vi "Accel Distance Calculator.vi"(11 "G-Input":dbl) -> (3 "Distance gone":dbl)   [LabVIEW 2014]
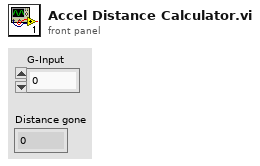
[diagram p1: front panel]
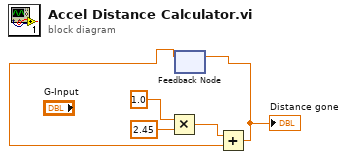
[diagram p0: block diagram]
diagram:
  n1 = Multiply(x=1.0, y=2.45) -> (x*y=w4:dbl)
  n2 = feedback #1() -> (w1:dbl)  [unwired: 1 in]
  n3 = Add(x=w4, y=w1) -> (x+y=w2:dbl)
  "Distance gone" <- w2
  n4 = feedback-in #1(w2) -> ()
